vi "PhysiologyExperiment_1file.vi"() -> ()   [LabVIEW 2017]
doc: "I. Description:\nThis example demonstrates how to continuously acquire and generate data at the same time, synchronized with one another.\n\nII. Instructions for Running:\n1. Select the physical channel to correspond to where your signal is input on the DAQ device. Also, select the corresponding channel for where your signal is being generated.\n2. Enter the minimum and maximum voltage ranges.\nNote: For better accuracy try to match the input range to the expected voltage level of the measured signal.\n3. Set the sample rate of the acquisition.\nNote: The rate should be at least twice as fast as the maximum frequency component of the signal being acquired. \n4. Select the Rate for the generation\n5. Select what type of signal to generate and the amplitude.\nNote: This example requires two DMA channels to run. If your hardware does not support two DMA channels, you need to set the Data Transfer Mechanism property for the Analog Output Task to use \"Interrupts\". The Data Transfer Mechanism property is located in the DAQmx Channel Property hierarchy at: DAQmx Channel Property Node>>Analog Output>>General Properties>>Advanced>>Data Transfer and Memory>>Data Transfer Mechanism\n\nRefer to your device documentation to determine how many DMA channels are supported for your hardware.\n\nIII. Block Diagram Steps:\n1. Create an analog input voltage channel. Also, create an analog output voltage channel.\n2. Set the rate for the sample clock. Additionally, define the sample mode to be continuous. Also, set the sample clock rate for the signal generation.\n2a. Call the Get Terminal Name with Device Prefix VI. This will take a Task and a terminal and create a properly formatted device + terminal name to use as the source of the Trigger.\n3. Define the parameters for a Digital Edge Start Trigger. Set the Analog output to trigger off the AI Start Trigger. This is an internal trigger signal.\n4. Use the Basic Function Generator VI to create the signal to be generated.\n5. Call the Start VI to arm the two functions. Make sure the analog output is armed before the analog input. This will ensure both will start at the same time.\n6. Read the waveform data in a loop until the user hits the stop button or an error occurs. The Is Task Done? VI is used to check for errors in the Analog Output Task.\n7. Call the Clear VI to Clear the Task\n8. Use the popup dialog box to display an error if any.\n\nIV. I/O Connections Overview:\nMake sure your signal input/output terminals match the Physical Channel I/O controls."
uses:
  <vilib>/Utility/error.llb/DialogType.ctl
  <vilib>/DAQmx/write.llb/DAQmx Write (Digital Wfm 1Chan NSamp).vi
  <vilib>/DAQmx/write.llb/DAQmx Write (Analog 1D Wfm NChan NSamp).vi
  <vilib>/DAQmx/miscellaneous.llb/DAQmx Fill In Error Info.vi
  <vilib>/Waveform/DWDTOps.llb/DWDT Uncompress Digital.vi
  <vilib>/DAQmx/configure/timing.llb/DAQmx Timing (Sample Clock).vi
  <vilib>/DAQmx/create/channels.llb/DAQmx Create Channel (DO-Digital Output).vi
  <vilib>/DAQmx/configure/trigger.llb/DAQmx Start Trigger (Digital Edge).vi
  <vilib>/DAQmx/create/channels.llb/DAQmx Create Channel (AO-Voltage-Basic).vi
  <vilib>/Waveform/DWDTOps.llb/DWDT Analog to Digital.vi
  <vilib>/Waveform/WDTOps.llb/WDT Number of Waveform Samples DBL.vi
  <resource>/objmgr/daqmx.rc
panel:
  in  "4k High-pass":bool=TRUE
  in  "Multiplier":dbl=1.0
  in  "Stimulus File":path=path "C:/data/Auditory/stim/strstim.wav"
  out "Stimulus overview":waveform(dbl)[](graph)
  out "Digital Waveform Graph":digitalwaveform(graph) caption="TTL Pulses"
  out "Actual Update Generation Rate":dbl=5000.0 format="%0.2f"
  out "Actual Input Rate":dbl=10000.0 format="%0.2f"
  in  "rate":dbl=500000.0 caption="Analog Output Update Rate" format="%0.2f"
  in  "minimum value":dbl=-10.0 caption="Output Minimum Value" format="%0.2f"
  in  "maximum value":dbl=10.0 caption="Output Maximum Value" format="%0.2f"
  in  "physical channels":tag="Dev1/ao0:1" caption="Analog Output Physical Channel"
  in  "Physical Channel":tag="Dev1/port0/line0" caption="Digital Output Physical Channel"
  in  "Rate":dbl=500000.0 caption="Digital Output Update Rate" format="%0.2f"
  in  "stop":bool
  # "Overview: This VI Generates Synchronized 2ch auditory stimulation and synchronization pulses\nRequirements: \nSoftware: LabVIEW 2012 (or compatible). The digital port need to support buffered operations (port 0 on PCIe-6341)\nInstructions: \n1.\tSelect the physical channels for the digital and analog outputs.\n2.\tEnter the minimum and maximum voltage ranges. \n3.\tSet the sample rate of the data generation. \n4.\tChoose the stimulus wave file that contains 3 ch (2 ch audio and TTL Pulses)  (16-bit integer wav only)\n5. Press start to start the stimulus"
  # "Output Channel Parameters"
  # "Timing Parameters"
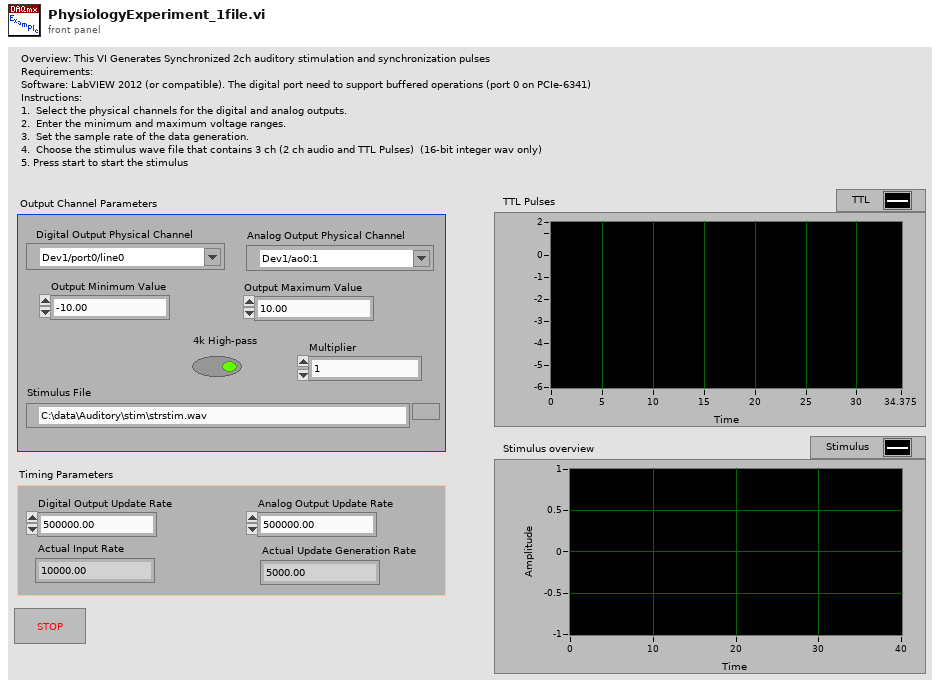
[diagram p1: front panel]
types:
  T1 = typedef "DialogType.ctl" = u16
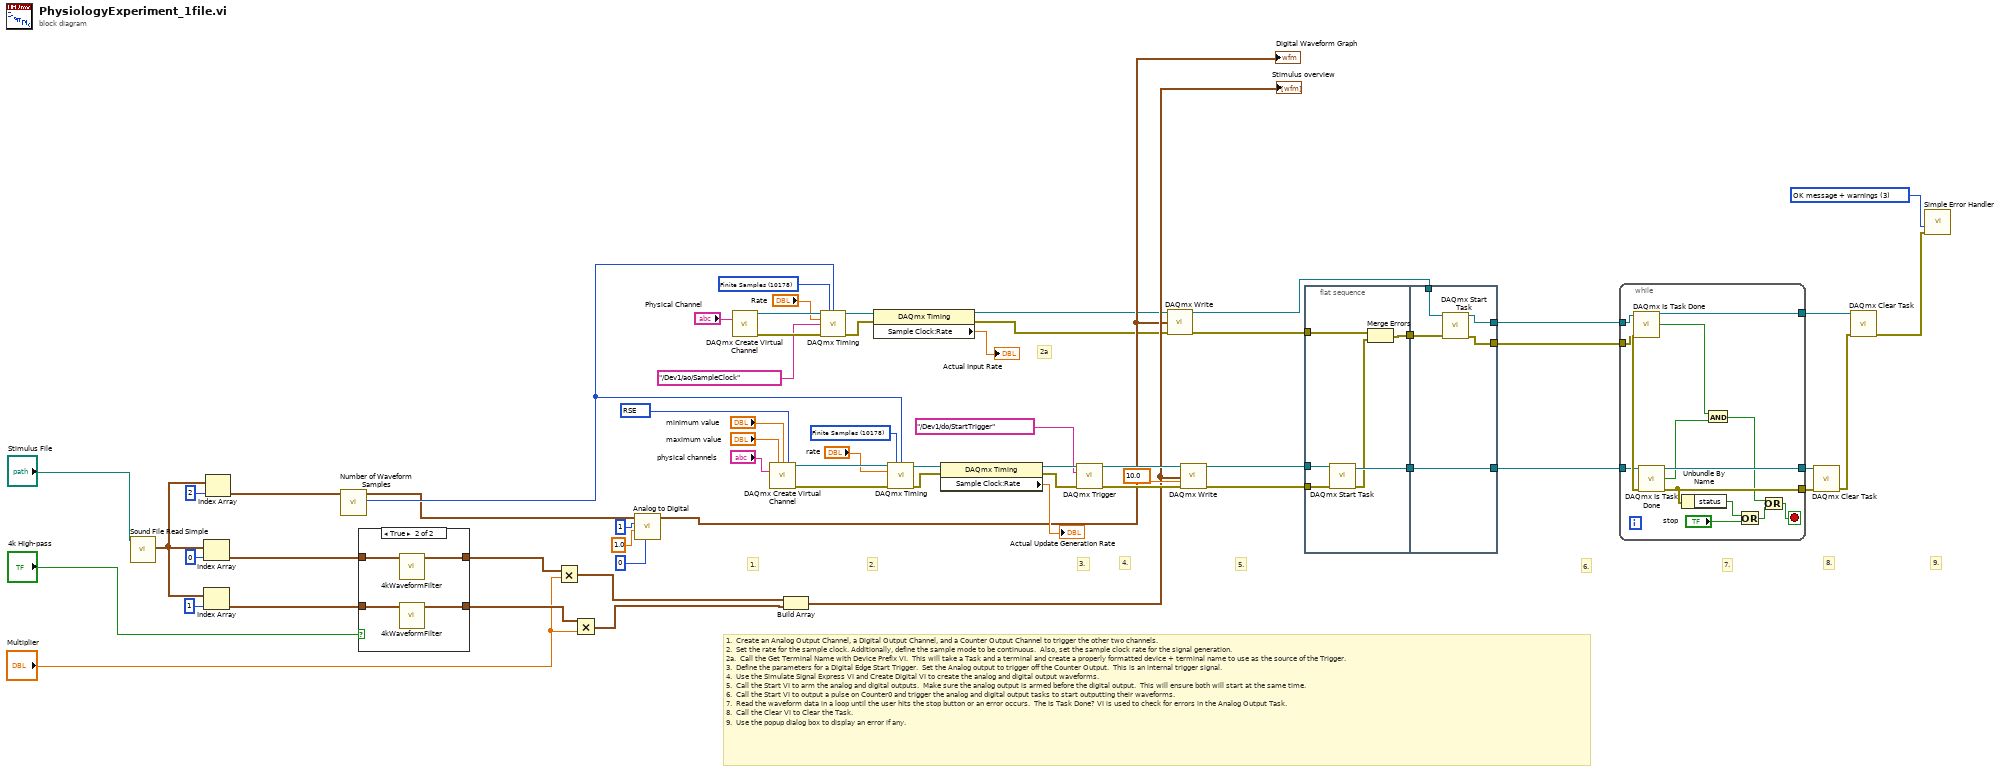
[diagram p0: block diagram]
diagram:
  w3 = 10083 items=["Default"=-1, "RSE"=10083, "Differential"=10106, "Pseudodifferential"=12529] ("output terminal configuration")
  w45 = T1 3 items=["no dialog", "OK message", "continue or stop message", "OK message + warnings", "continue/stop + warnings"] ("type of dialog (OK msg:1)")
  w57 = 10178 items=["Finite Samples"=10178, "Continuous Samples"=10123] ("sample mode")
  w63 = 10178 items=["Finite Samples"=10178, "Continuous Samples"=10123] ("sample mode")
  # "9."
  # "2a"
  # "6."
  # "3."
  # "4."
  # "8."
  # "5."
  # "7."
  # "1.  Create an Analog Output Channel, a Digital Output Channel, and a Counter Output Channel to trigger the other two channels.\n2.  Set the rate for the sample clock. Additionally, define the sample mode to be continuous.  Also, set the sample clock rate for the signal generation.\n2a.  Call the Get Terminal Name with Device Prefix VI.  This will take a Task and a terminal and create a properly formatted device + terminal name to use as the source of the Trigger.\n3.  Define the parameters for a Digital Edge Start Trigger.  Set the Analog output to trigger off the Counter Output.  This is an internal trigger signal.\n4.  Use the Simulate Signal Express VI and Create Digital VI to create the analog and digital output waveforms.\n5.  Call the Start VI to arm the analog and digital outputs.  Make sure the analog output is armed before the digital output.  This will ensure both will start at the same time.\n6.  Call the Start VI to output a pulse on Counter0 and trigger the analog and digital output tasks to start outputting their waveforms.\n7.  Read the waveform data in a loop until the user hits the stop button or an error occurs.  The Is Task Done? VI is used to check for errors in the Analog Output Task.\n8.  Call the Clear VI to Clear the Task.\n9.  Use the popup dialog box to display an error if any."
  # "2."
  # "1."
  n1 = call <vilib>:"Sound File Read Simple.vi"("path"="Stimulus File") -> ("data"=w28:waveform(dbl)[])  [unwired: 7 in, 3 out]
  n2 = Index Array(array=w28, index=0) -> (element=w24:waveform(dbl))
  n3 = Index Array(array=w28, index=1) -> (element=w20:waveform(dbl))
  n4 = Index Array(array=w28, index=2) -> (element=w5:waveform(dbl))
  n5 = call-poly <vilib>:"Number of Waveform Samples.vi"("waveform in"=w5) -> ("number of samples"=w13:i32, "waveform out"=w4:waveform(dbl))  [unwired: 8 in, 1 out]
  n6 = case shown="True" "4k High-pass" {
    tunnel: w24 -> [w66 w70]
    tunnel: [w66 w69] -> w18
    tunnel: [w65 w68] -> w16
    tunnel: w20 -> [w65 w67]
    frame False {
    }
    frame True {
      n7 = call "4kWaveformFilter.vi"("data"=w70) -> ("Waveform"=w69:waveform(dbl))  [unwired: 10 in]
      n8 = call "4kWaveformFilter.vi"("data"=w67) -> ("Waveform"=w68:waveform(dbl))  [unwired: 10 in]
    }
  }
  n9 = Multiply(x=w18, y="Multiplier") -> (x*y=w17:waveform(dbl))
  n10 = Multiply(x=w16, y="Multiplier") -> (x*y=w15:waveform(dbl))
  n11 = call-poly <vilib>:"Analog to Digital.vi"("data format (offset binary)"=0, "full-scale range (pk-pk)"=1.0, "resolution (16 bit)"=1, "analog waveform"=w4) -> ("digital waveform"=w22:digitalwaveform)  [unwired: 4 in, 3 out]
  "Digital Waveform Graph" <- w22
  n12 = call-poly <vilib>:"DAQmx Create Virtual Channel.vi"("lines"="Physical Channel") -> ("task out"=w61:refnum<k21>, "error out"=w62:errorcluster)  [unwired: 6 in, 7 out]
  n13 = call-poly <vilib>:"DAQmx Create Virtual Channel.vi"("maximum value"="maximum value", "minimum value"="minimum value", "output terminal configuration"=w3, "physical channels"="physical channels") -> ("task out"=w56:refnum<k21>, "error out"=w55:errorcluster)  [unwired: 5 in, 5 out]
  n14 = Build Array(w17, w15) -> (w23:waveform(dbl)[])
  "Stimulus overview" <- w23
  n15 = call-poly <vilib>:"DAQmx Timing.vi"("task/channels in"=w61, "sample mode"=w63, "samples per channel"=w13, "rate"="Rate", "source"=tag "/Dev1/ao/SampleClock", "error in"=w62) -> ("task out"=w38:refnum<k21>, "error out"=w32:errorcluster)  [unwired: 1 in, 7 out]
  n16 = property class="DAQmx Timing"(reference=w38, error in=w32) -> (reference out=w2:refnum<k21>, error out=w1:errorcluster, "Sample Clock:Rate"=→"Actual Input Rate":dbl)
  n17 = call-poly <vilib>:"DAQmx Timing.vi"("task/channels in"=w56, "sample mode"=w57, "samples per channel"=w13, "rate"="rate", "error in"=w55) -> ("task out"=w42:refnum<k21>, "error out"=w41:errorcluster)  [unwired: 2 in, 7 out]
  n18 = property class="DAQmx Timing"(reference=w42, error in=w41) -> (reference out=w43:refnum<k21>, error out=w40:errorcluster, "Sample Clock:Rate"=→"Actual Update Generation Rate":dbl)
  n19 = call-poly <vilib>:"DAQmx Trigger.vi"("task/channels in"=w43, "source"=tag "/Dev1/do/StartTrigger", "error in"=w40) -> ("task out"=w47:refnum<k21>, "error out"=w48:errorcluster)  [unwired: 2 in, 9 out]
  n20 = call-poly <vilib>:"DAQmx Write.vi"("task/channels in"=w2, "data"=w22, "error in"=w1) -> ("task out"=w8:refnum<k21>, "error out"=w33:errorcluster)  [unwired: 2 in, 9 out]
  n21 = call-poly <vilib>:"DAQmx Write.vi"("task/channels in"=w47, "data"=w23, "timeout"=10.0 ("Wirite Timeout"), "error in"=w48) -> ("task out"=w50:refnum<k21>, "error out"=w49:errorcluster)  [unwired: 1 in, 9 out]
  n22 = flat-sequence {
    tunnel: w50 -> [w75]
    tunnel: w49 -> [w74]
    tunnel: w33 -> [w71]
    tunnel: [w76] -> w10
    tunnel: [w72] -> w9
    tunnel: [w81] -> w54
    tunnel: w10 -> [w81]
    tunnel: w9 -> [w79]
    tunnel: w8 -> [w80]
    tunnel: [w78] -> w7
    tunnel: [w77] -> w6
    frame #0 {
      n23 = call <vilib>:"DAQmx Start Task.vi"("task/channels in"=w75, "error in"=w74) -> ("task out"=w76:refnum<k21>, "error out"=w73:errorcluster)  [unwired: 12 out]
      n24 = Merge Errors(w71, w73) -> (w72:errorcluster)
    }
    frame #1 {
      n25 = call <vilib>:"DAQmx Start Task.vi"("task/channels in"=w80, "error in"=w79) -> ("task out"=w78:refnum<k21>, "error out"=w77:errorcluster)  [unwired: 12 out]
    }
  }
  n26 = while {
    tunnel: [w95] -> w64
    tunnel: w54 -> [w91]
    tunnel: [w90] -> w53
    tunnel: [w89] -> w36
    tunnel: w7 -> [w83]
    tunnel: w6 -> [w82]
    stop <- w84 stop-if-true
    n27 = call <vilib>:"DAQmx Is Task Done.vi"("task/channels in"=w83, "error in"=w82) -> ("task out"=w95:refnum<k21>, "task done?"=w88:bool, "error out"=w92:errorcluster)  [unwired: 2 in, 9 out]
    n28 = call <vilib>:"DAQmx Is Task Done.vi"("task/channels in"=w91, "error in"=w92) -> ("task out"=w90:refnum<k21>, "task done?"=w87:bool, "error out"=w89:errorcluster)  [unwired: 11 out]
    n29 = Unbundle By Name(w89) -> ("status"=w93:bool)
    n30 = And(x=w88, y=w87) -> (x .and. y?=w86:bool)
    n31 = Or(x=w93, y="stop") -> (x .or. y?=w85:bool)
    n32 = Or(x=w86, y=w85) -> (x .or. y?=w84:bool)
  }
  n33 = call <vilib>:"DAQmx Clear Task.vi"("task in"=w53, "error in"=w36) -> ("error out"=w35:errorcluster)  [unwired: 13 out]
  n34 = call <vilib>:"DAQmx Clear Task.vi"("task in"=w64, "error in"=w35) -> ("error out"=w11:errorcluster)  [unwired: 13 out]
  n35 = call <vilib>:"Simple Error Handler.vi"("type of dialog (OK msg:1)"=w45, "error in (no error)"=w11) -> ()  [unwired: 3 in, 5 out]
